vi "PCO_ImageTiming.vi"() -> (0 "PCO_ImageTiming":T2, 1 "PCO_ImageTiming_Raw":T1, 2 "Length":u16, 3 "Raw_Length":u16)   [LabVIEW 2019, in "SDK.lvlib" / "Structures.lvlib"]
doc: "Use this template to build a VI to use as a subVI."
uses:
  Structures.lvlib
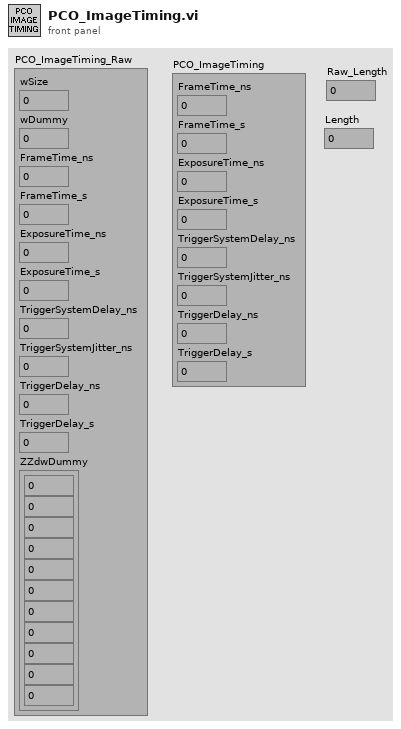
[diagram p1: front panel]
types:
  T1 = cluster{"wSize":u16, "wDummy":u16, "FrameTime_ns":u32, "FrameTime_s":u32, "ExposureTime_ns":u32, "ExposureTime_s":u32, "TriggerSystemDelay_ns":u32, "TriggerSystemJitter_ns":u32, "TriggerDelay_ns":u32, "TriggerDelay_s":u32, "ZZdwDummy":cluster{u32, u32, u32, u32, u32, u32, u32, u32, u32, u32, u32}}
  T2 = cluster{"FrameTime_ns":u32, "FrameTime_s":u32, "ExposureTime_ns":u32, "ExposureTime_s":u32, "TriggerSystemDelay_ns":u32, "TriggerSystemJitter_ns":u32, "TriggerDelay_ns":u32, "TriggerDelay_s":u32}
  T3 = cluster{u32, u32, u32, u32, u32, u32, u32, u32, u32, u32, u32}
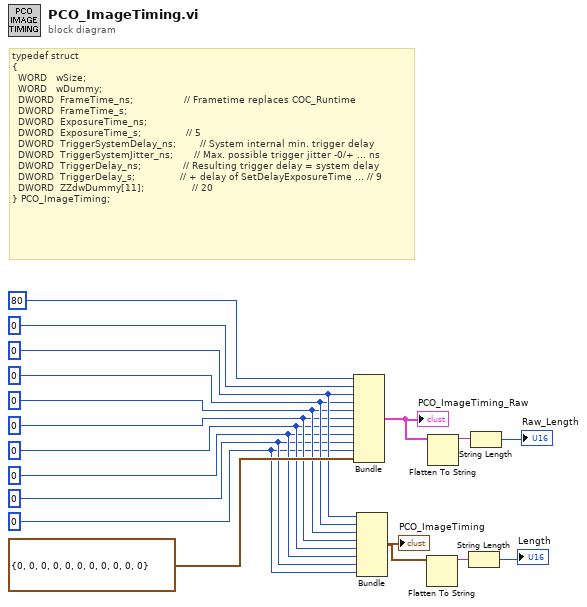
[diagram p0: block diagram]
diagram:
  w1 = u32 0 ("TriggerDelay_s")
  w2 = u32 0 ("TriggerDelay_ns")
  w3 = u32 0 ("TriggerSystemJitter_ns")
  w4 = u32 0 ("TriggerSystemDelay_ns")
  w5 = u32 0 ("ExposureTime_s")
  w6 = u32 0 ("ExposureTime_ns")
  w7 = u32 0 ("FrameTime_s")
  w8 = u32 0 ("FrameTime_ns")
  # "typedef struct\n{\n  WORD   wSize;\n  WORD   wDummy;\n  DWORD  FrameTime_ns;                 // Frametime replaces COC_Runtime\n  DWORD  FrameTime_s;   \n  DWORD  ExposureTime_ns;\n  DWORD  ExposureTime_s;               // 5\n  DWORD  TriggerSystemDelay_ns;        // System internal min. trigger delay\n  DWORD  TriggerSystemJitter_ns;       // Max. possible trigger jitter -0/+ ... ns\n  DWORD  TriggerDelay_ns;              // Resulting trigger delay = system delay\n  DWORD  TriggerDelay_s;               // + delay of SetDelayExposureTime ... // 9\n  DWORD  ZZdwDummy[11];                // 20\n} PCO_ImageTiming;"
  n1 = Bundle("wSize"=u16 80, "wDummy"=u16 0, "FrameTime_ns"=w8, "FrameTime_s"=w7, "ExposureTime_ns"=w6, "ExposureTime_s"=w5, "TriggerSystemDelay_ns"=w4, "TriggerSystemJitter_ns"=w3, "TriggerDelay_ns"=w2, "TriggerDelay_s"=w1, "ZZdwDummy"=T3 {0, 0, 0, 0, 0, 0, 0, 0, 0, 0, 0}) -> (w11:T1)  [unwired: 1 in]
  "PCO_ImageTiming_Raw" <- w11
  n2 = Bundle("FrameTime_ns"=w8, "FrameTime_s"=w7, "ExposureTime_ns"=w6, "ExposureTime_s"=w5, "TriggerSystemDelay_ns"=w4, "TriggerSystemJitter_ns"=w3, "TriggerDelay_ns"=w2, "TriggerDelay_s"=w1) -> (w17:T2)  [unwired: 1 in]
  "PCO_ImageTiming" <- w17
  n3 = Flatten To String(anything=w17) -> (data string=w16:string)  [unwired: 3 in, 2 out]
  n4 = Flatten To String(anything=w11) -> (data string=w15:string)  [unwired: 3 in, 2 out]
  n5 = String Length(string=w16) -> (length=→"Length":i32)
  n6 = String Length(string=w15) -> (length=→"Raw_Length":i32)
